vi "vipm_target_version.vi"() -> (3 "vipm Taget version":string)   [LabVIEW 2017, in "_Try Beta Version of CSMF.lvlib"]
uses:
  _Try Beta Version of CSMF.lvlib
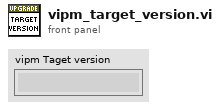
[diagram p1: front panel]
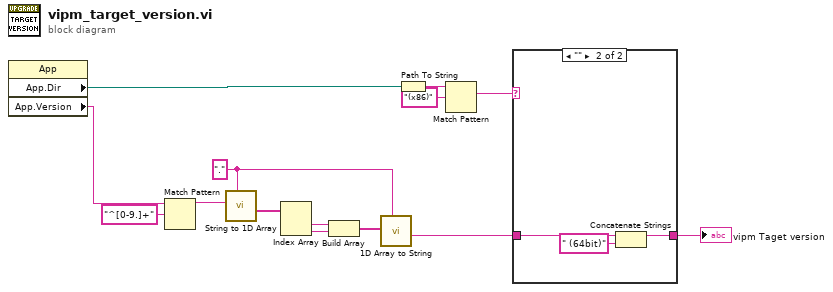
[diagram p0: block diagram]
diagram:
  w10 = "." ("delimiter (Tab)")
  n1 = property class="App"() -> ("App.Dir"=w9:path, "App.Version"=w2:string)  [unwired: 2 in, 2 out]
  n2 = Match Pattern(string=w2, regular expression="^[0-9.]+") -> (match substring=w3:string)  [unwired: 1 in, 3 out]
  n3 = call "String to 1D Array.vi"("delimiter (Tab)"=w10, "string"=w3) -> ("Array of Strings"=w14:string[])  [unwired: 9 in]
  n4 = Index Array(array=w14) -> (element #1=w12:string, element #2=w13:string)  [unwired: 2 in]
  n5 = Build Array(w12, w13) -> (w11:string[])
  n6 = call "1D Array to String.vi"("delimiter (Tab)"=w10, "Array of Strings"=w11) -> ("delimited string"=w5:string)  [unwired: 9 in]
  n7 = Path To String(path=w9) -> (string=w8:string)
  n8 = Match Pattern(string=w8, regular expression="(x86)") -> (match substring=w6:string)  [unwired: 1 in, 3 out]
  n9 = case shown="\"\"" w6 {
    tunnel: [w15 w17] -> w4
    tunnel: w5 -> [w15 w18]
    frame Default {
    }
    frame "" {
      n10 = Concatenate Strings(w18, " (64bit)" ("string")) -> (w17:string)
    }
  }
  "vipm Taget version" <- w4
